vi "Actor.vi"(6 "Host Name":string, 7 "Transport Queue":refnum<queue>, 8 "error in (no error)":errorcluster, 9 "Actor Name":string, 10 "Message Broker Interface":refnum<class "Message Broker Interface.lvclass">, 11 "Mediated Asynchronous Actor in":refnum<class "Mediated Asynchronous Actor.lvclass">) -> (0 "error out":errorcluster, 3 "Mediated Asynchronous Actor out":refnum<class "Mediated Asynchronous Actor.lvclass">)   [LabVIEW 2016, in "Stream Mediator.lvlib" / "Mediated Asynchronous Actor.lvclass"]
doc: "--\nCopyright © 2017 Composed SystemsI All rights reserved.\n\nAuthor: Jon McBee <jon.mcbee@composed.io>\n\nThis library is provided \"AS IS\" ,WITHOUT WARRANTIES OR\nCONDITIONS OF ANY KIND, either express or implied.\n\nComposed Systems -- composed.io\n\nStream 0.0.1.1\nJon McBee - Composed Systems\nCopyright (c) 2017, Composed Systems"
uses:
  <userlib>/Composed Systems/Stream/Mediator/Classes/Mediated Asynchronous Actor/Mediated Asynchronous Actor.lvclass
  C:/Program Files (x86)/National Instruments/LabVIEW 2016/user.lib/Composed Systems/Stream/Mediator/Classes/Mediated Actor/Mediated Actor.lvclass
  <userlib>/Composed Systems/Stream/Mediator/Classes/Message Broker Interface/Message Broker Interface.lvclass
  <userlib>/Composed Systems/Stream/Mediator/Classes/Message Transport Interface/Message Transport Interface.lvclass
  <userlib>/Composed Systems/Stream/Mediator/Classes/Mediated Asynchronous Actor/Mediated Asynchronous Actor.lvclass/Mediated Asynchronous Actor.ctl
  <userlib>/Composed Systems/Stream/Mediator/Classes/Message Transport Queue/Message Transport Queue.lvclass
  C:/Program Files (x86)/National Instruments/LabVIEW 2016/user.lib/Composed Systems/Stream/Mediator/Classes/Message Transport Interface/Message Transport Interface.lvclass
  <userlib>/Composed Systems/Stream/Mediator/Classes/Message Command Last Ack/Last Ack.lvclass
  <userlib>/Composed Systems/Stream/Mediator/Classes/Mediated Actor/Mediated Actor.lvclass
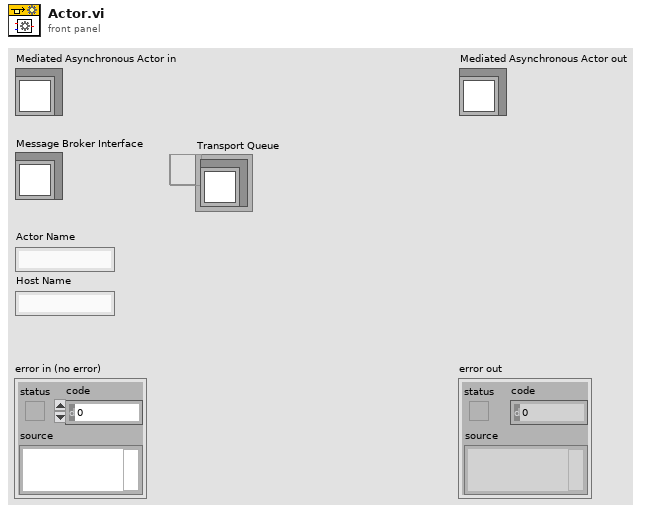
[diagram p1: front panel]
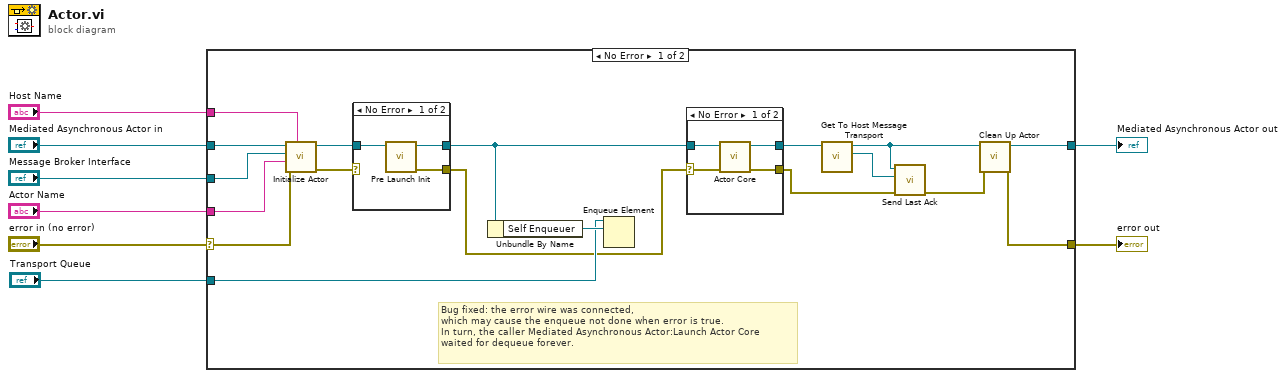
[diagram p0: block diagram]
diagram:
  n1 = case shown="No Error" "error in (no error)" {
    selector: "error in (no error)" -> [w22 w39]
    tunnel: [w10 w39] -> w7
    tunnel: [w16 w38] -> w5
    tunnel: "Mediated Asynchronous Actor in" -> [w26 w38]
    tunnel: "Message Broker Interface" -> [w25 _]
    tunnel: "Host Name" -> [w24 _]
    tunnel: "Actor Name" -> [w23 _]
    tunnel: "Transport Queue" -> [w18 _]
    frame No Error {
      # "Bug fixed: the error wire was connected,\nwhich may cause the enqueue not done when error is true.\nIn turn, the caller Mediated Asynchronous Actor:Launch Actor Core\nwaited for dequeue forever."
      n2 = call-dynamic "Initialize Actor.vi"("Host Name"=w24, "error in (no error)"=w22, "Actor Name"=w23, "Message Broker Interface"=w25, "Mediated Asynchronous Actor in"=w26) -> ("error out"=w20:errorcluster, "Mediated Asynchronous Actor out"=w21:refnum<class "Mediated Asynchronous Actor.lvclass">)  [unwired: 5 in]
      n3 = case shown="No Error" w20 {
        selector: w20 -> [_ w37]
        tunnel: w21 -> [w35 w36]
        tunnel: [w34 w36] -> w17
        tunnel: [w33 w37] -> w9
        frame No Error {
          n4 = call-dynamic "Pre Launch Init.vi"("Mediated Asynchronous Actor in"=w35) -> ("error out"=w33:errorcluster, "Mediated Asynchronous Actor out"=w34:refnum<class "Mediated Asynchronous Actor.lvclass">)  [unwired: 9 in]
        }
        frame Error {
        }
      }
      n5 = Unbundle By Name(w17) -> ("Self Enqueuer"=w19:refnum<class "Message Transport Queue.lvclass">)
      n6 = Enqueue Element(queue=w18, element=w19) -> ()  [unwired: 2 in, 3 out]
      n7 = case shown="No Error" w9 {
        selector: w9 -> [w29 w31]
        tunnel: w17 -> [w30 w32]
        tunnel: [w28 w32] -> w15
        tunnel: [w27 w31] -> w12
        frame No Error {
          n8 = call-dynamic "Actor Core.vi"("error in (no error)"=w29, "Mediated Asynchronous Actor in"=w30) -> ("error out"=w27:errorcluster, "Mediated Asynchronous Actor out"=w28:refnum<class "Mediated Asynchronous Actor.lvclass">)  [unwired: 8 in]
        }
        frame Error {
        }
      }
      n9 = call <userlib>:"Get To Host Message Transport.vi"("Mediated Actor in"=w15) -> ("To Host"=w14:refnum<class "Message Transport Queue.lvclass">, "Mediated Actor out"=w13:refnum<class "Mediated Asynchronous Actor.lvclass">)  [unwired: 9 in]
      n10 = call <userlib>:"Send Last Ack.vi"("error in (no error)"=w12, "Message Transport Queue in"=w14, "Mediated Asynchronous Actor"=w13) -> ("error out"=w11:errorcluster)  [unwired: 8 in]
      n11 = call-dynamic "Clean Up Actor.vi"("error in (no error)"=w11, "Mediated Asynchronous Actor in"=w13) -> ("error out"=w10:errorcluster, "Mediated Asynchronous Actor out"=w16:refnum<class "Mediated Asynchronous Actor.lvclass">)  [unwired: 8 in]
    }
    frame Error {
    }
  }
  "error out" <- w7
  "Mediated Asynchronous Actor out" <- w5
